vi "Brass_1.vi"(0 "Amount":fxp<+,8,0>, 8 "Gate":bool, 10 "M":fxp<+,32,32>, 11 "Trigger":bool) -> (3 "Brass Out":fxp<+/-,8,8>)   [LabVIEW 2015]
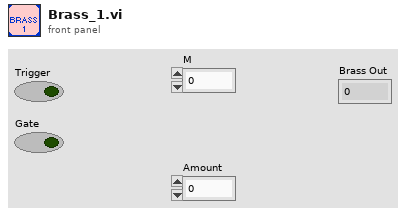
[diagram p1: front panel]
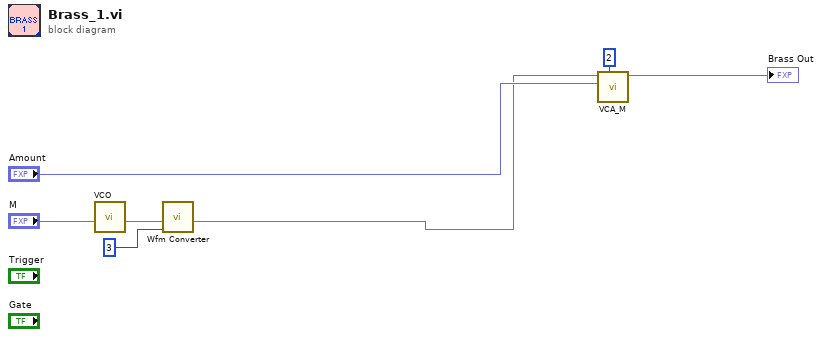
[diagram p0: block diagram]
diagram:
  n1 = call "VCO.vi"("M"="M") -> ("Sine Sample"=w4:fxp<+/-,8,8>)  [unwired: 10 in]
  n2 = call "Wfm Converter.vi"("Select"=u8 3 ("select"), "Sample In"=w4) -> ("Sample Out"=w1:fxp<+/-,8,8>)  [unwired: 9 in]
  n3 = call "VCA_M.vi"("Scale"=i8 2, "Amount"="Amount", "Sample In"=w1) -> ("Sample Out"=→"Brass Out":fxp<+/-,8,8>)  [unwired: 8 in]
